vi "tictock.vi"(8 "error in (no error)":errorcluster, 11 "seconds since 1Jan1904 2":timestamp) -> (0 "error out":errorcluster, 2 "Numeric":dbl, 3 "seconds since 1Jan1904":timestamp)   [LabVIEW 2018]
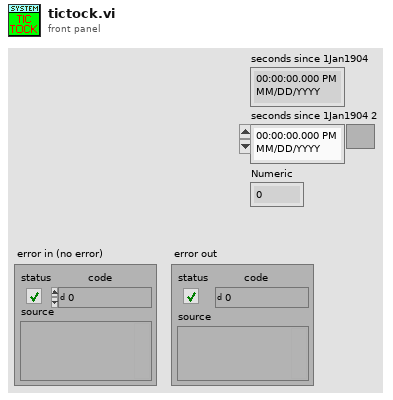
[diagram p1: front panel]
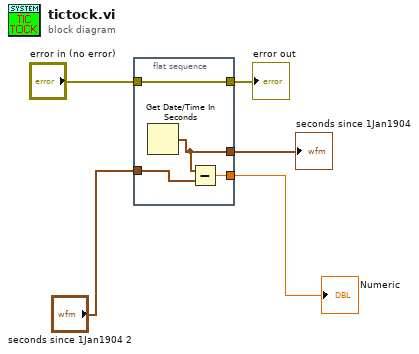
[diagram p0: block diagram]
diagram:
  n1 = flat-sequence {
    tunnel: [w6] -> w5
    tunnel: "seconds since 1Jan1904 2" -> [w9]
    tunnel: [w8] -> w1
    tunnel: "error in (no error)" -> [w7]
    tunnel: [w7] -> w3
    frame #0 {
      n2 = Get Date/Time In Seconds() -> (seconds since 1Jan1904=w6:timestamp)
      n3 = Subtract(x=w6, y=w9) -> (x-y=w8:dbl)
    }
  }
  "error out" <- w3
  "seconds since 1Jan1904" <- w5
  "Numeric" <- w1
